vi "HEWH Gas Thermal Raw Calc.vi"(0 "Input Data":T1, 11 "error in (no error)":errorcluster) -> (4 "Rate":dbl, 6 "Eff":dbl format="%#.5g", 8 "Gallons (Gal)":dbl, 10 "Gas Mass Flow":dbl, 15 "error out":errorcluster)   [LabVIEW 2020]
uses:
  Thermal Calculation Cluster.ctl
  HEWH Water Properties.ctl
panel:
  out "Density (lb/gal)":dbl format="%#.9g"
  out "Specific Heat (BTU/lbm*F)":dbl
  out "RTDout":dbl
  out "B":dbl
  out "A":dbl
  out "Heat input":dbl
  # "Debug Data"
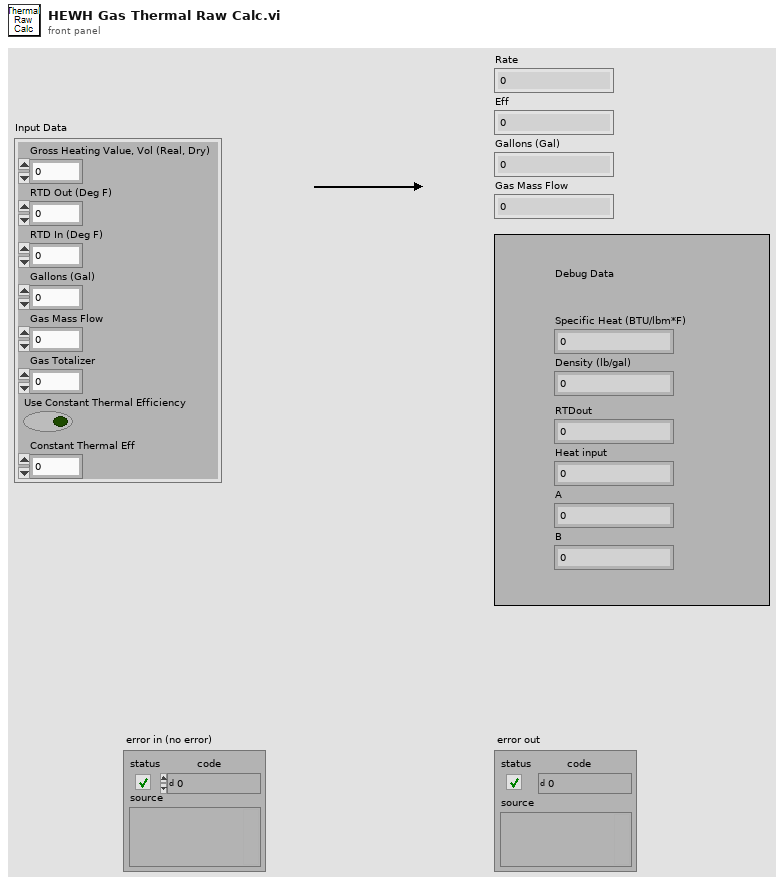
[diagram p1: front panel]
types:
  T1 = typedef "Thermal Calculation Cluster.ctl" = cluster{"Gross Heating Value, Vol (Real, Dry)":dbl, "RTD Out (Deg F)":dbl, "RTD In (Deg F)":dbl, "Gallons (Gal)":dbl, "Gas Mass Flow":dbl, "Gas Totalizer":dbl, "Use Constant Thermal Efficiency":bool, "Constant Thermal Eff":dbl}
  T2 = typedef "HEWH Water Properties.ctl" = enum16{"GEA Intertek Values", "CSA Values", "ANSI Values"}
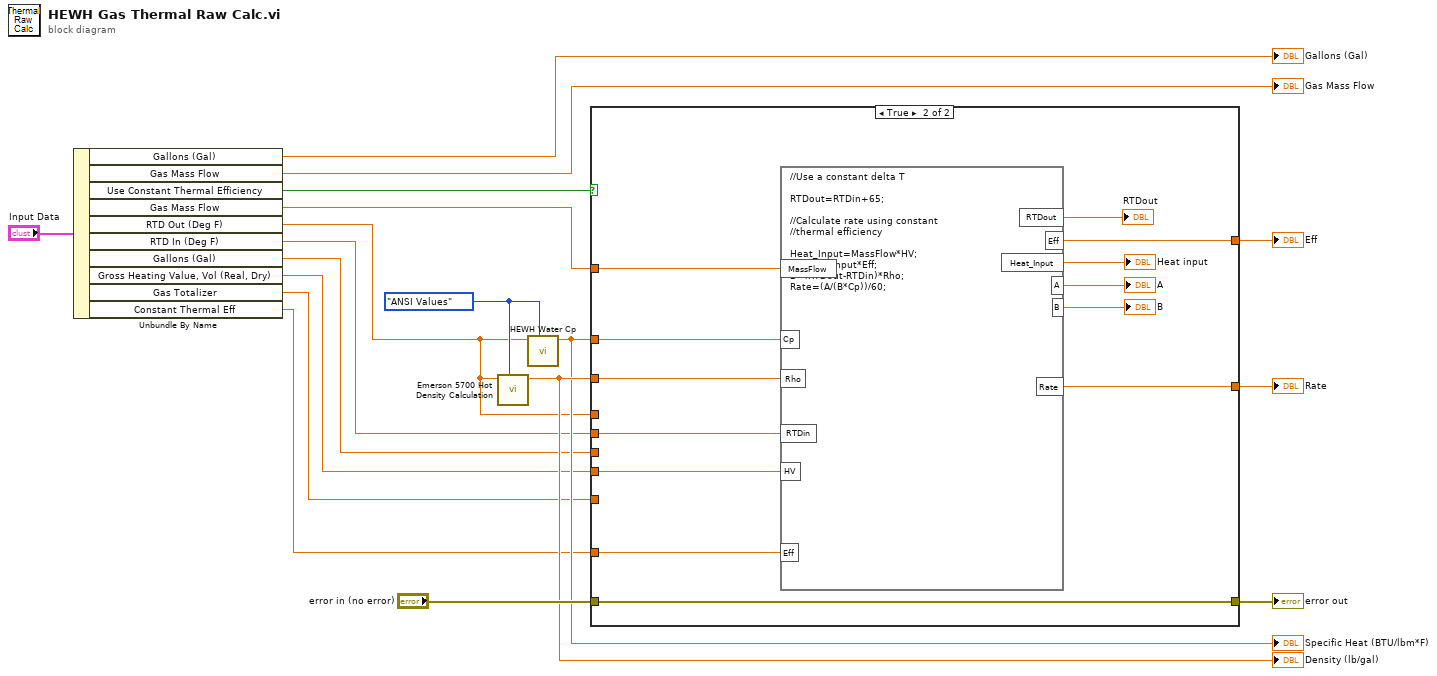
[diagram p0: block diagram]
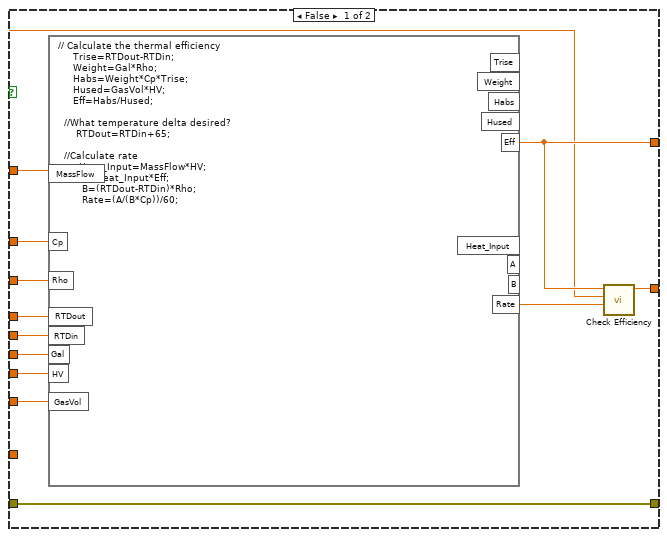
[diagram p2: hidden frame]
diagram:
  w14 = HEWH_Water_Properties."ANSI Values" ("Water Properties Reference")
  n1 = Unbundle By Name("Input Data") -> ("Gallons (Gal)"=→"Gallons (Gal)":dbl, "Gas Mass Flow"=→"Gas Mass Flow":dbl, "Use Constant Thermal Efficiency"=w10:bool, "Gas Mass Flow"=w9:dbl, "RTD Out (Deg F)"=w8:dbl, "RTD In (Deg F)"=w7:dbl, "Gallons (Gal)"=w6:dbl, "Gross Heating Value, Vol (Real, Dry)"=w5:dbl, "Gas Totalizer"=w4:dbl, "Constant Thermal Eff"=w3:dbl)
  n2 = call "Emerson 5700 Hot Density Calculation.vi"("Water Properties Reference"=w14, "RTD Out (°F)"=w8) -> ("Density (lb/gal)"=w16:dbl)  [unwired: 8 in, 1 out]
  "Density (lb/gal)" <- w16
  n3 = call "HEWH Water Cp.vi"("Water Properties Reference"=w14, "Input Temperature (°F)"=w8) -> ("Specific Heat (BTU/lbm*F)"=w15:dbl)  [unwired: 8 in, 1 out]
  "Specific Heat (BTU/lbm*F)" <- w15
  n4 = case shown="True" w10 {
    tunnel: [w30 w43] -> w18
    tunnel: "error in (no error)" -> [w30 w43]
    tunnel: w8 -> [w25 _]
    tunnel: w16 -> [w29 w38]
    tunnel: w15 -> [w28 w39]
    tunnel: w7 -> [w27 w42]
    tunnel: w5 -> [w26 w41]
    tunnel: w9 -> [w21 w40]
    tunnel: [w22 w37] -> w13
    tunnel: [w24 w33] -> w12
    tunnel: w6 -> [w20 _]
    tunnel: w4 -> [w19 _]
    tunnel: w3 -> [_ w31]
    frame False {
      n5 = formula code="// Calculate the thermal efficiency\n     Trise=RTDout-RTDin;\n     Weight=Gal*Rho;\n     Habs=Weight*Cp*Trise;\n     Hused=GasVol*HV;\n     Eff=Habs/Hused;\n\n  //What temperature delta desired?\n      RTDout=RTDin+65;\n          \n  //Calculate rate\n       Heat_Input=MassFlow*HV;\n        A=Heat_Input*Eff;\n        B=(RTDout-RTDin)*Rho;\n        Rate=(A/(B*Cp))/60;"("RTDin"=w27, "MassFlow"=w21, "Gal"=w20, "GasVol"=w19, "HV"=w26, "Cp"=w28, "Rho"=w29, "RTDout"=w25) -> ("Rate"=w23:dbl, "Eff"=w24:dbl)  [unwired: 7 out]
      n6 = call "Check Efficiency.vi"("Rate"=w23, "Gas Mass Flow"=w21, "Eff"=w24) -> ("Adjuste Rate"=w22:dbl)  [unwired: 8 in]
    }
    frame True {
      n7 = formula code="//Use a constant delta T\n\nRTDout=RTDin+65;\n\n//Calculate rate using constant\n//thermal efficiency\n\nHeat_Input=MassFlow*HV;\nA=Heat_Input*Eff;\nB=(RTDout-RTDin)*Rho;\nRate=(A/(B*Cp))/60;"("RTDin"=w42, "MassFlow"=w40, "HV"=w41, "Cp"=w39, "Rho"=w38, "Eff"=w31) -> ("Rate"=w37:dbl, "Heat_Input"=→"Heat input":dbl, "A"=→"A":dbl, "B"=→"B":dbl, "Eff"=w33:dbl, "RTDout"=→"RTDout":dbl)
    }
  }
  "error out" <- w18
  "Rate" <- w13
  "Eff" <- w12
